vi "getFilterHeadingSource.vi"(8 "error in (no error)":errorcluster, 11 "pHandle":u32) -> (0 "error out":errorcluster, 2 "return type":i32, 3 "headingSourceStr":string)   [LabVIEW 2011, in "sbgLabView.lvlib"]
uses:
  sbgLabView.lvlib
  sbgMatLab.dll
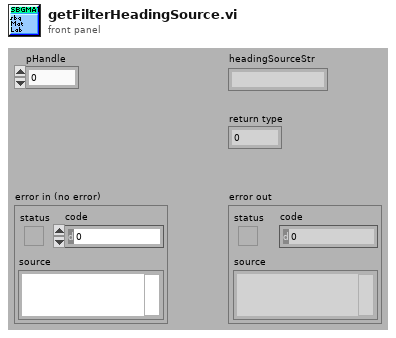
[diagram p1: front panel]
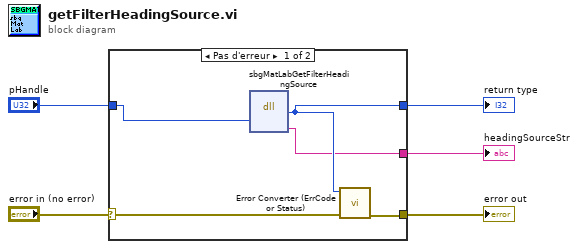
[diagram p0: block diagram]
diagram:
  n1 = case shown="Pas d'erreur" "error in (no error)" {
    selector: "error in (no error)" -> [w7 w11]
    tunnel: [w6 w11] -> w4
    tunnel: [w10 _] -> w3
    tunnel: "pHandle" -> [w9 _]
    tunnel: [w8 _] -> w1
    frame No Error {
      n2 = dll-call lib="C:/SBG-Systems/remote/projects/software/projects/labviewExample/sbgLabView/sbgMatLab.*" fn="sbgMatLabGetFilterHeadingSource"("pHandle"=w9) -> ("return type"=w10:i32, "sourceStr"=w8:string)  [unwired: 5 in, 2 out]
      n3 = call "Error Converter (ErrCode or Status).vi"("error in (no error)"=w7, "error code"=w10) -> ("error out"=w6:errorcluster)  [unwired: 9 in]
    }
    frame Error {
    }
  }
  "return type" <- w3
  "headingSourceStr" <- w1
  "error out" <- w4
